vi "sendMessage.vi"(8 "error in (no error)":errorcluster, 10 "message":string, 11 "MonoCommunicator in":refnum<class "MonoCommunicator.lvclass">) -> (0 "error out":errorcluster, 3 "MonoCommunicator out":refnum<class "MonoCommunicator.lvclass">)   [LabVIEW 2016, in "MonoCommunicator.lvclass"]
uses:
  MonoCommunicator.lvclass
  MonoCommunicator.lvclass/MonoCommunicator.ctl
  ts_labview_tcp/TCPCommunicator/TCPCommunicator.lvclass/TCPCommunicator.ctl
  ts_labview_tcp/TCPServer/TCPServer.lvclass
  C:/Users/aanania/Documents/ts_monochromator_windows/ts_labview_tcp/TCPCommunicator/TCPCommunicator.lvclass
  ts_labview_tcp/TCPComEvents/TCPComEvents.lvclass
  ts_labview_tcp/TCPCommunicator/TCPCommunicator.lvclass
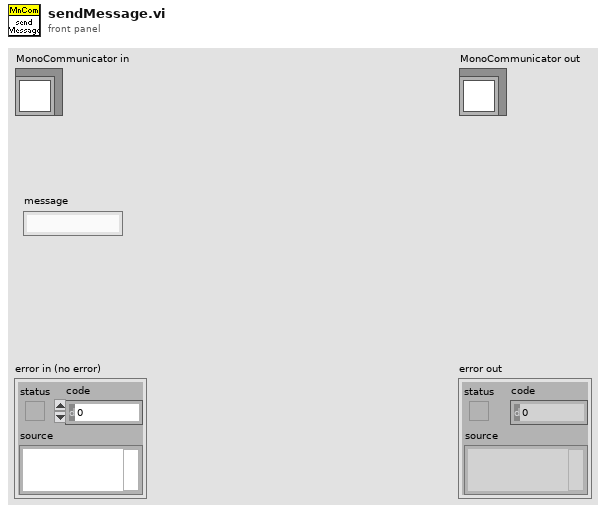
[diagram p1: front panel]
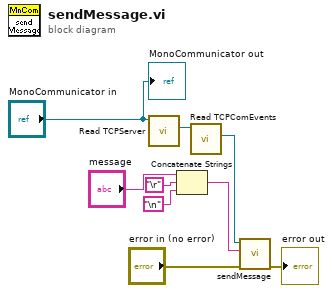
[diagram p0: block diagram]
diagram:
  n1 = call "Read TCPServer.vi"("MonoCommunicator in"="MonoCommunicator in") -> ("TCPServer.lvclass"=w3:refnum<class "TCPServer.lvclass">)  [unwired: 8 in, 2 out]
  n2 = Concatenate Strings("message", "\r", "\n") -> (w1:string)
  n3 = call "Read TCPComEvents.vi"("TCPCommunicator in"=w3) -> ("TCPComEvents.lvclass"=w2:refnum<class "TCPComEvents.lvclass">)  [unwired: 8 in, 2 out]
  n4 = call "sendMessage.vi"("error in (no error)"="error in (no error)", "message"=w1, "TCPComEvents in"=w2) -> ("error out"=→"error out":errorcluster)  [unwired: 7 in, 1 out]
  "MonoCommunicator out" <- "MonoCommunicator in"
